vi "insert.vi"(5 "add line break after?":bool=TRUE, 7 "add line break before?":bool, 8 "error in (no error)":errorcluster, 10 "string":string, 11 "Notebook in":refnum<class "Notebook.lvclass">) -> (0 "error out":errorcluster, 3 "Notebook out":refnum<class "Notebook.lvclass">)   [LabVIEW 2010, in "Notebook.lvclass"]
uses:
  Notebook.lvclass
  Notebook.lvclass/Notebook.ctl
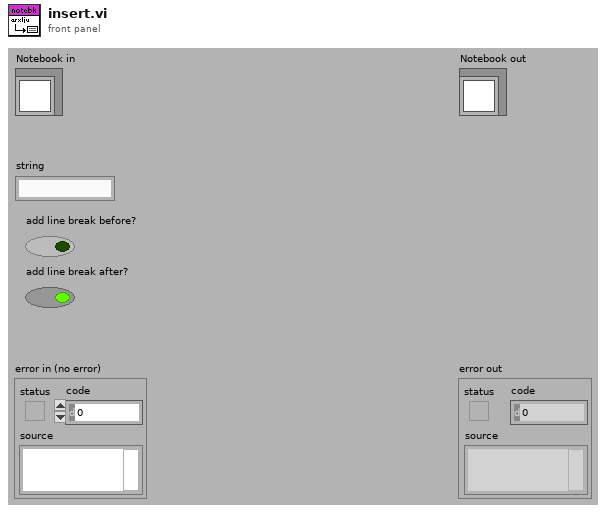
[diagram p1: front panel]
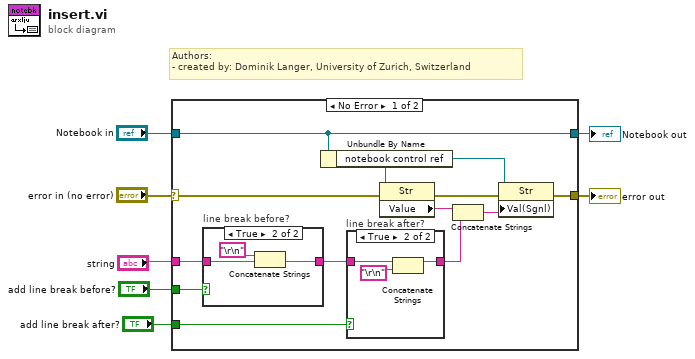
[diagram p0: block diagram]
diagram:
  # "Authors: \n- created by: Dominik Langer, University of Zurich, Switzerland"
  n1 = case shown="No Error" "error in (no error)" {
    selector: "error in (no error)" -> [w16 w29]
    tunnel: [w18 w29] -> w6
    tunnel: [w19 w28] -> w4
    tunnel: "Notebook in" -> [w19 w28]
    tunnel: "string" -> [w10 _]
    tunnel: "add line break after?" -> [w11 _]
    tunnel: "add line break before?" -> [w8 _]
    frame No Error {
      n2 = case "line break before?" shown="True" w8 {
        tunnel: w10 -> [w20 w23]
        tunnel: [w20 w21] -> w9
        frame False {
        }
        frame True {
          n3 = Concatenate Strings("\r\n", w23) -> (w21:string)
        }
      }
      n4 = Unbundle By Name(w19) -> ("notebook control ref"=w17:refnum<vi>)
      n5 = case "line break after?" shown="True" w11 {
        tunnel: w9 -> [w24 w27]
        tunnel: [w24 w26] -> w12
        frame False {
        }
        frame True {
          n6 = Concatenate Strings(w27, "\r\n") -> (w26:string)
        }
      }
      n7 = property class="Str"(reference=w17, error in=w16) -> (error out=w15:errorcluster, "Value"=w14:string)  [unwired: 1 out]
      n8 = Concatenate Strings(w14, w12) -> (w13:string)
      n9 = property class="Str"(reference=w17, error in=w15, "Val(Sgnl)"=w13) -> (error out=w18:errorcluster)  [unwired: 1 out]
    }
    frame Error {
    }
  }
  "error out" <- w6
  "Notebook out" <- w4
